vi "GET_MAC.vi"(8 "error in (no error)":errorcluster) -> (0 "error out":errorcluster, 2 "array":string[][](array[string]), 3 "MAC":string)   [LabVIEW 2017]
panel:
  out "subarray":string[](array[string])
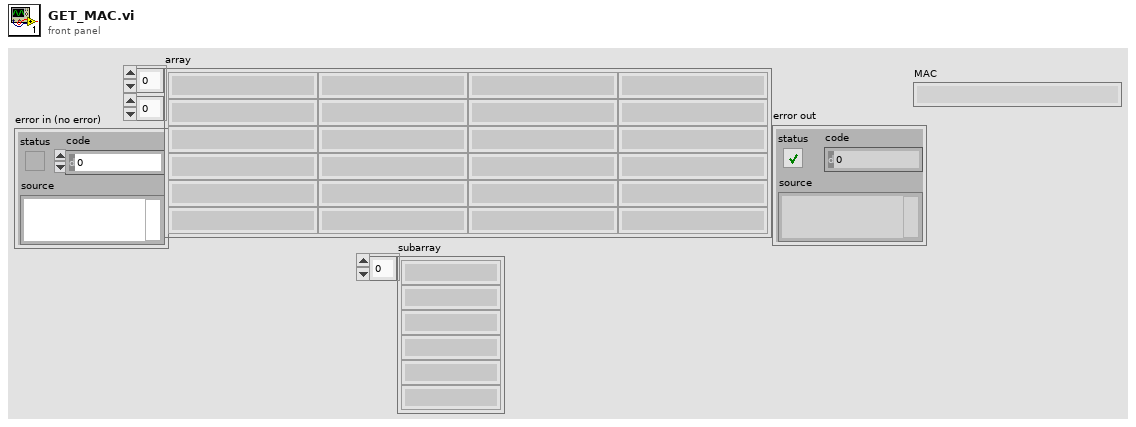
[diagram p1: front panel]
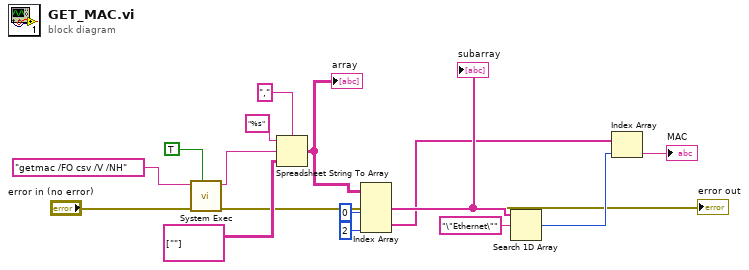
[diagram p0: block diagram]
diagram:
  n1 = call <vilib>:"System Exec.vi"("wait until completion? (T)"=TRUE ("run minimized? (F)"), "error in (no error)"="error in (no error)", "command line"="getmac /FO csv /V /NH") -> ("error out"=→"error out":errorcluster, "standard output"=w11:string)  [unwired: 5 in, 2 out]
  n2 = Spreadsheet String To Array(delimiter (Tab)=",", format string="%s", spreadsheet string=w11, array type (2D Dbl)=string[][] [[""]]) -> (array=w6:string[][])
  "array" <- w6
  n3 = Index Array(array=w6, index (col) #1=0 ("disabled index (col)"), index (col) #2=2 ("index (col)")) -> (element #1=w8:string[], element #2=w4:string[])  [unwired: 2 in]
  "subarray" <- w8
  n4 = Search 1D Array(1D array=w8, element="\"Ethernet\"") -> (index of element=w3:i32)  [unwired: 1 in]
  n5 = Index Array(array=w4, index=w3) -> (element=→"MAC":string)
